vi "Info from Folder.vi"(8 "error in (no error)":errorcluster, 9 "Name":string, 10 "Folder":path, 11 "GitPackage in":refnum<class "GitPackage.lvclass">) -> (0 "error out":errorcluster, 2 "Package Info":T1)   [LabVIEW 2020, in "GPack.lvlib" / "GitPackage.lvclass"]
uses:
  GitPackage.lvclass
  Package Info.ctl
  <vilib>/Hampel Software Engineering/Git API/Git API/GIT-api.lvclass/GIT-api.ctl
  <vilib>/Hampel Software Engineering/Git API/Git API/GIT-api.lvclass
  GPack.lvlib
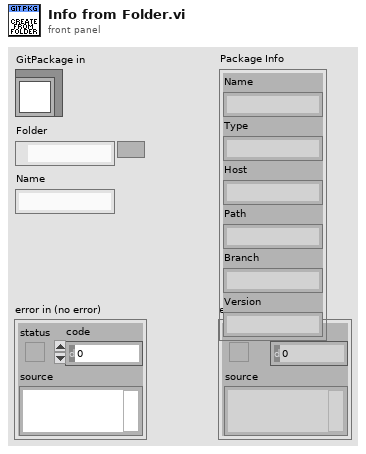
[diagram p1: front panel]
types:
  T1 = typedef "GPack.lvlib/Package Info.ctl" = cluster{"Name":string, "Type":string, "Host":string, "Path":string, "Branch":string, "Version":string}
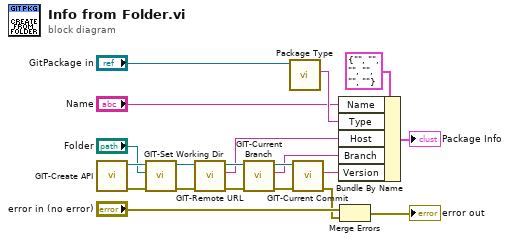
[diagram p0: block diagram]
diagram:
  n1 = call <vilib>:"GIT-Create API.vi"() -> ("error out"=w20:errorcluster, "git-api out"=w18:refnum<class "GIT-api.lvclass">)  [unwired: 10 in]
  n2 = call <vilib>:"GIT-Set Working Dir.vi"("error in"=w20, "Working Directory"="Folder", "git-api in"=w18) -> ("error out"=w10:errorcluster, "git-api out"=w11:refnum<class "GIT-api.lvclass">)  [unwired: 7 in]
  n3 = call <vilib>:"GIT-Remote URL.vi"("error in"=w10, "git-api in"=w11) -> ("error out"=w9:errorcluster, "remote url"=w7:string, "git-api out"=w8:refnum<class "GIT-api.lvclass">)  [unwired: 7 in]
  n4 = call <vilib>:"GIT-Current Branch.vi"("error in"=w9, "git-api in"=w8) -> ("error out"=w15:errorcluster, "current branch"=w6:string, "git-api out"=w16:refnum<class "GIT-api.lvclass">)  [unwired: 6 in, 1 out]
  n5 = call-dynamic "Package Type.vi"("GitPackage in"="GitPackage in") -> ("Type"=w13:string)  [unwired: 9 in, 1 out]
  n6 = call <vilib>:"GIT-Current Commit.vi"("error in"=w15, "git-api in"=w16) -> ("error out"=w1:errorcluster, "current commit"=w5:string)  [unwired: 7 in, 1 out]
  n7 = Bundle By Name(cluster=T1 {"Name"="", "Type"="", "Host"="", "Path"="", "Branch"="", "Version"=""} ("Package Info"), "Name"="Name", "Type"=w13, "Host"=w7, "Branch"=w6, "Version"=w5) -> (→"Package Info":T1)
  n8 = Merge Errors("error in (no error)", w1) -> (→"error out":errorcluster)
